vi "总氮通讯.vi"() -> ()   [LabVIEW 2016, in "斯坦道总氮.lvlib"]
uses:
  <vilib>/NI/Modbus Library/API/Wrapper/Create TCP Slave.vi
  <vilib>/Utility/config.llb/Write Key (Boolean).vi
  <vilib>/Utility/config.llb/Write Key (String).vi
  <vilib>/Plasmionique/MB Master/MB_Master/MB_Master.lvclass
  <vilib>/NI/Modbus Library/API/Slave/Modbus Slave.lvclass
  <vilib>/Utility/config.llb/NI_LVConfig.lvlib
  <vilib>/Plasmionique/MB Master/MB Master.lvlib
  <vilib>/NI/Modbus Library/API/Wrapper/API Main.lvlib
panel:
  out "总氮测量数据区":u16[](array[numeric])
  out "总氮状态告警区":u16[](array[numeric])
  out "总磷状态告警区":u16[](array[numeric])
  out "总磷测量数据区":u16[](array[numeric])
  out "序列号":string
  out "状态告警区":T1 {"告警代码" items=["无告警", "缺试剂告警", "缺水样告警", "缺蒸馏水告警", "缺标液告警", "仪表漏液告警", "标定异常告警", "超量程告警", "加热异常", "低试剂预警", "超上限告警", "超下限告警", "仪表内部其他异常", "滴定异常告警", "电极异常告警", "量程切换告警", "参数设置告警", "PH电极电位异常", "电导率电极异常", "浊度光度异常", "溶解氧电极异常", "溶解氧光强异常", "温度异常告警", "PH异常告警", "溶解氧异常告警", "电导率异常告警", "浊度异常告警", "叶绿素异常告警", "藻密度异常告警", "蓝绿藻异常告警", "ORP异常告警", "氨氮异常告警", "清洁刷异常告警", "SD卡异常告警", "蓝牙异常告警", "Wifi异常告警", "流程异常告警"]; "故障代码" items=["无故障", "电机故障", "温度故障", "通讯故障", "滴定故障"]}
  out "测量数据区":T2 {"单位" items=["ug/L", "mg/L", "ppm", "mg/m3", "cm", "ppb", "ug/m3", "%", "nmol/mol", "umol/mol", "MPN/L", "MPN/100ml", "ng/m3", "NTU", "无量纲", "ms/cm", "us/cm", "℃", "mV", "万个/L"]}
  out "status":bool
  out "关键参数区":T3
  in  "读关键参数区":bool
  in  "读状态告警区":bool
  in  "读测量数据区":bool
  in  "站号":u16(ring) items=["总磷"=1, "氨氮"=3]
  in  "停止":bool
  in  "启动":bool
  in  "控制命令":u16(ring) items=["启动测量"=1, "标样核查"=2, "零点核查"=3, "跨度核查"=4, "空白测试"=5, "平行样测试"=6, "加标回收"=7, "空白校准"=8, "标样校准"=9, "初始化（清洗）"=10, "停止测试"=11, "仪器重启"=12, "校时"=13, "模式设置"=14, "测量间隔设置"=15]
  in  "控制命令参数":u16[](array[numeric]) format="%04xH"
  in  "VISA Resource":refnum<visa-resource-name>
  in  "启用模块":bool
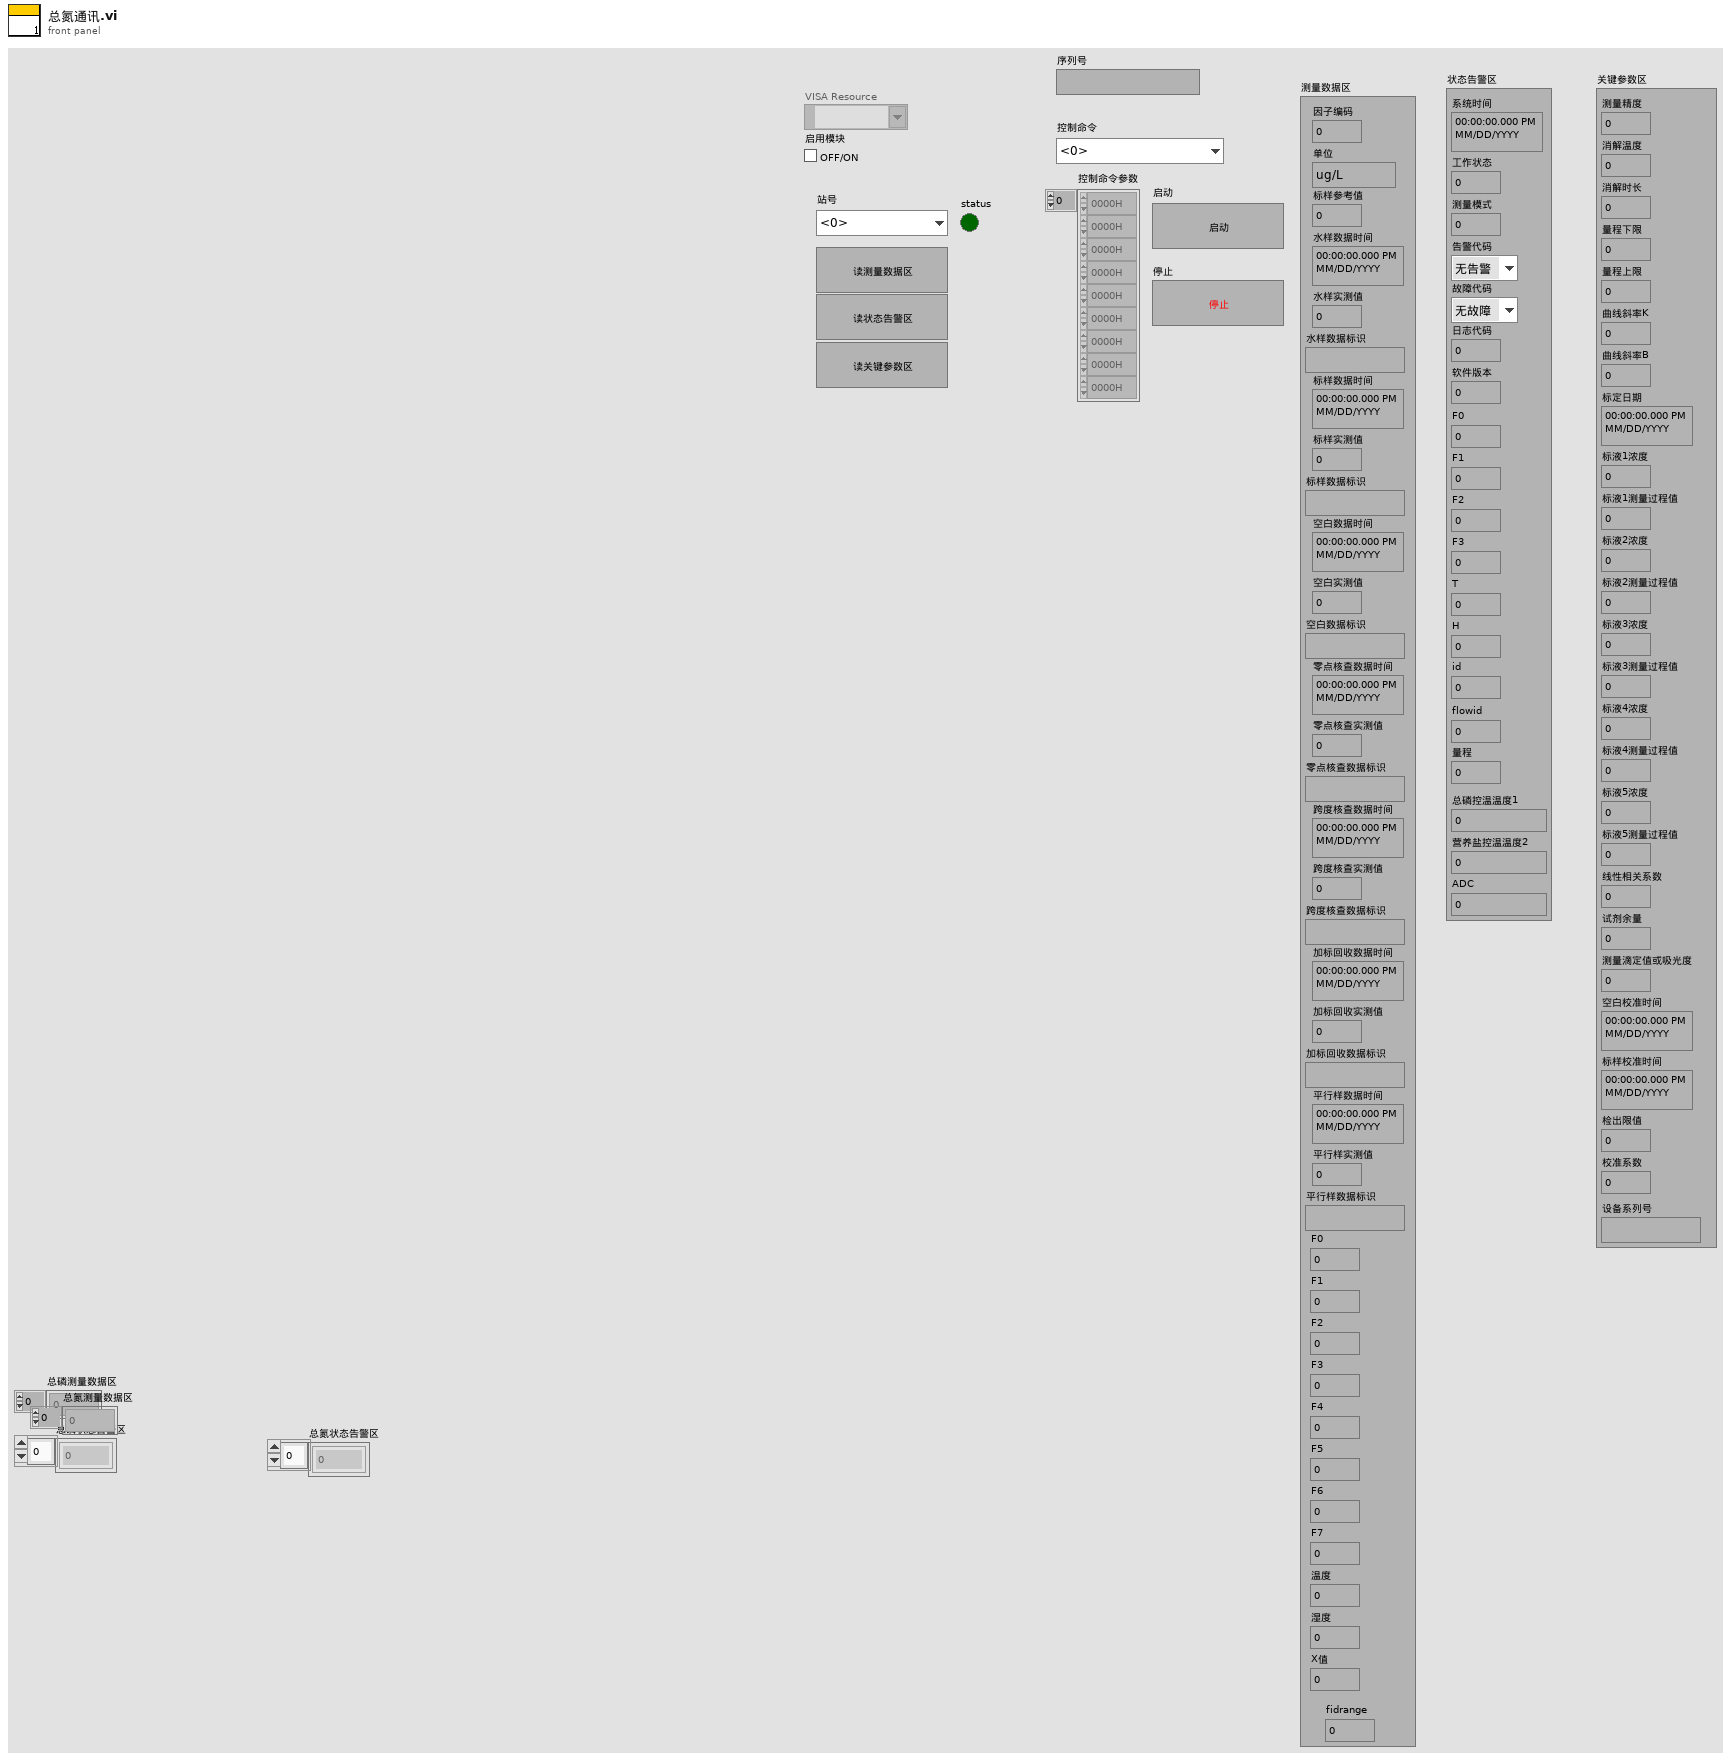
[diagram p1: front panel]
types:
  T1 = cluster{"系统时间":timestamp, "工作状态":u16, "测量模式":u16, "告警代码":u16, "故障代码":u16, "日志代码":u16, "软件版本":u16, "F0":sgl, "F1":sgl, "F2":sgl, "F3":sgl, "T":sgl, "H":sgl, "id":u16, "flowid":u16, "量程":u16, "总磷控温温度1":sgl, "营养盐控温温度2":sgl, "ADC":sgl}
  T2 = cluster{"因子编码":u32, "单位":u16, "标样参考值":sgl, "水样数据时间":timestamp, "水样实测值":sgl, "水样数据标识":string, "标样数据时间":timestamp, "标样实测值":sgl, "标样数据标识":string, "空白数据时间":timestamp, "空白实测值":sgl, "空白数据标识":string, "零点核查数据时间":timestamp, "零点核查实测值":sgl, "零点核查数据标识":string, "跨度核查数据时间":timestamp, "跨度核查实测值":sgl, "跨度核查数据标识":string, "加标回收数据时间":timestamp, "加标回收实测值":sgl, "加标回收数据标识":string, "平行样数据时间":timestamp, "平行样实测值":sgl, "平行样数据标识":string, "F0":sgl, "F1":sgl, "F2":sgl, "F3":sgl, "F4":sgl, "F5":sgl, "F6":sgl, "F7":sgl, "温度":sgl, "湿度":sgl, "X值":sgl, "fidrange":u16}
  T3 = cluster{"测量精度":u16, "消解温度":u16, "消解时长":u16, "量程下限":sgl, "量程上限":sgl, "曲线斜率K":sgl, "曲线斜率B":sgl, "标定日期":timestamp, "标液1浓度":sgl, "标液1测量过程值":sgl, "标液2浓度":sgl, "标液2测量过程值":sgl, "标液3浓度":sgl, "标液3测量过程值":sgl, "标液4浓度":sgl, "标液4测量过程值":sgl, "标液5浓度":sgl, "标液5测量过程值":sgl, "线性相关系数":sgl, "试剂余量":u32, "测量滴定值或吸光度":sgl, "空白校准时间":timestamp, "标样校准时间":timestamp, "检出限值":sgl, "校准系数":sgl, "设备系列号":string}
  T4 = typedef "NI_LVConfig.lvlib/Config Data RefNum.ctl" = refnum<k1>
  T5 = enum8{"Enabled", "Disabled", "Disabled and Grayed Out"}
  T6 = cluster{"系统时间":timestamp, "工作状态":enum16{"空闲", "水样测试", "标样核查", "零点核查", "跨度核查", "空白测试", "平行样测试", "加标回收", "空白校准", "标样校准", "初始化（清洗）"}, "测量模式":enum16{"待机", "连续模式", "周期模式", "定点模式", "受控模式", "手动模式"}, "告警代码":u16, "故障代码":u16, "日志代码":u16, "软件版本":u16, "F0":sgl, "F1":sgl, "F2":sgl, "F3":sgl, "T":sgl, "H":sgl, "id":u16, "flowid":u16, "量程":u16, "总磷控温温度1":sgl, "营养盐控温温度2":sgl, "ADC":sgl}
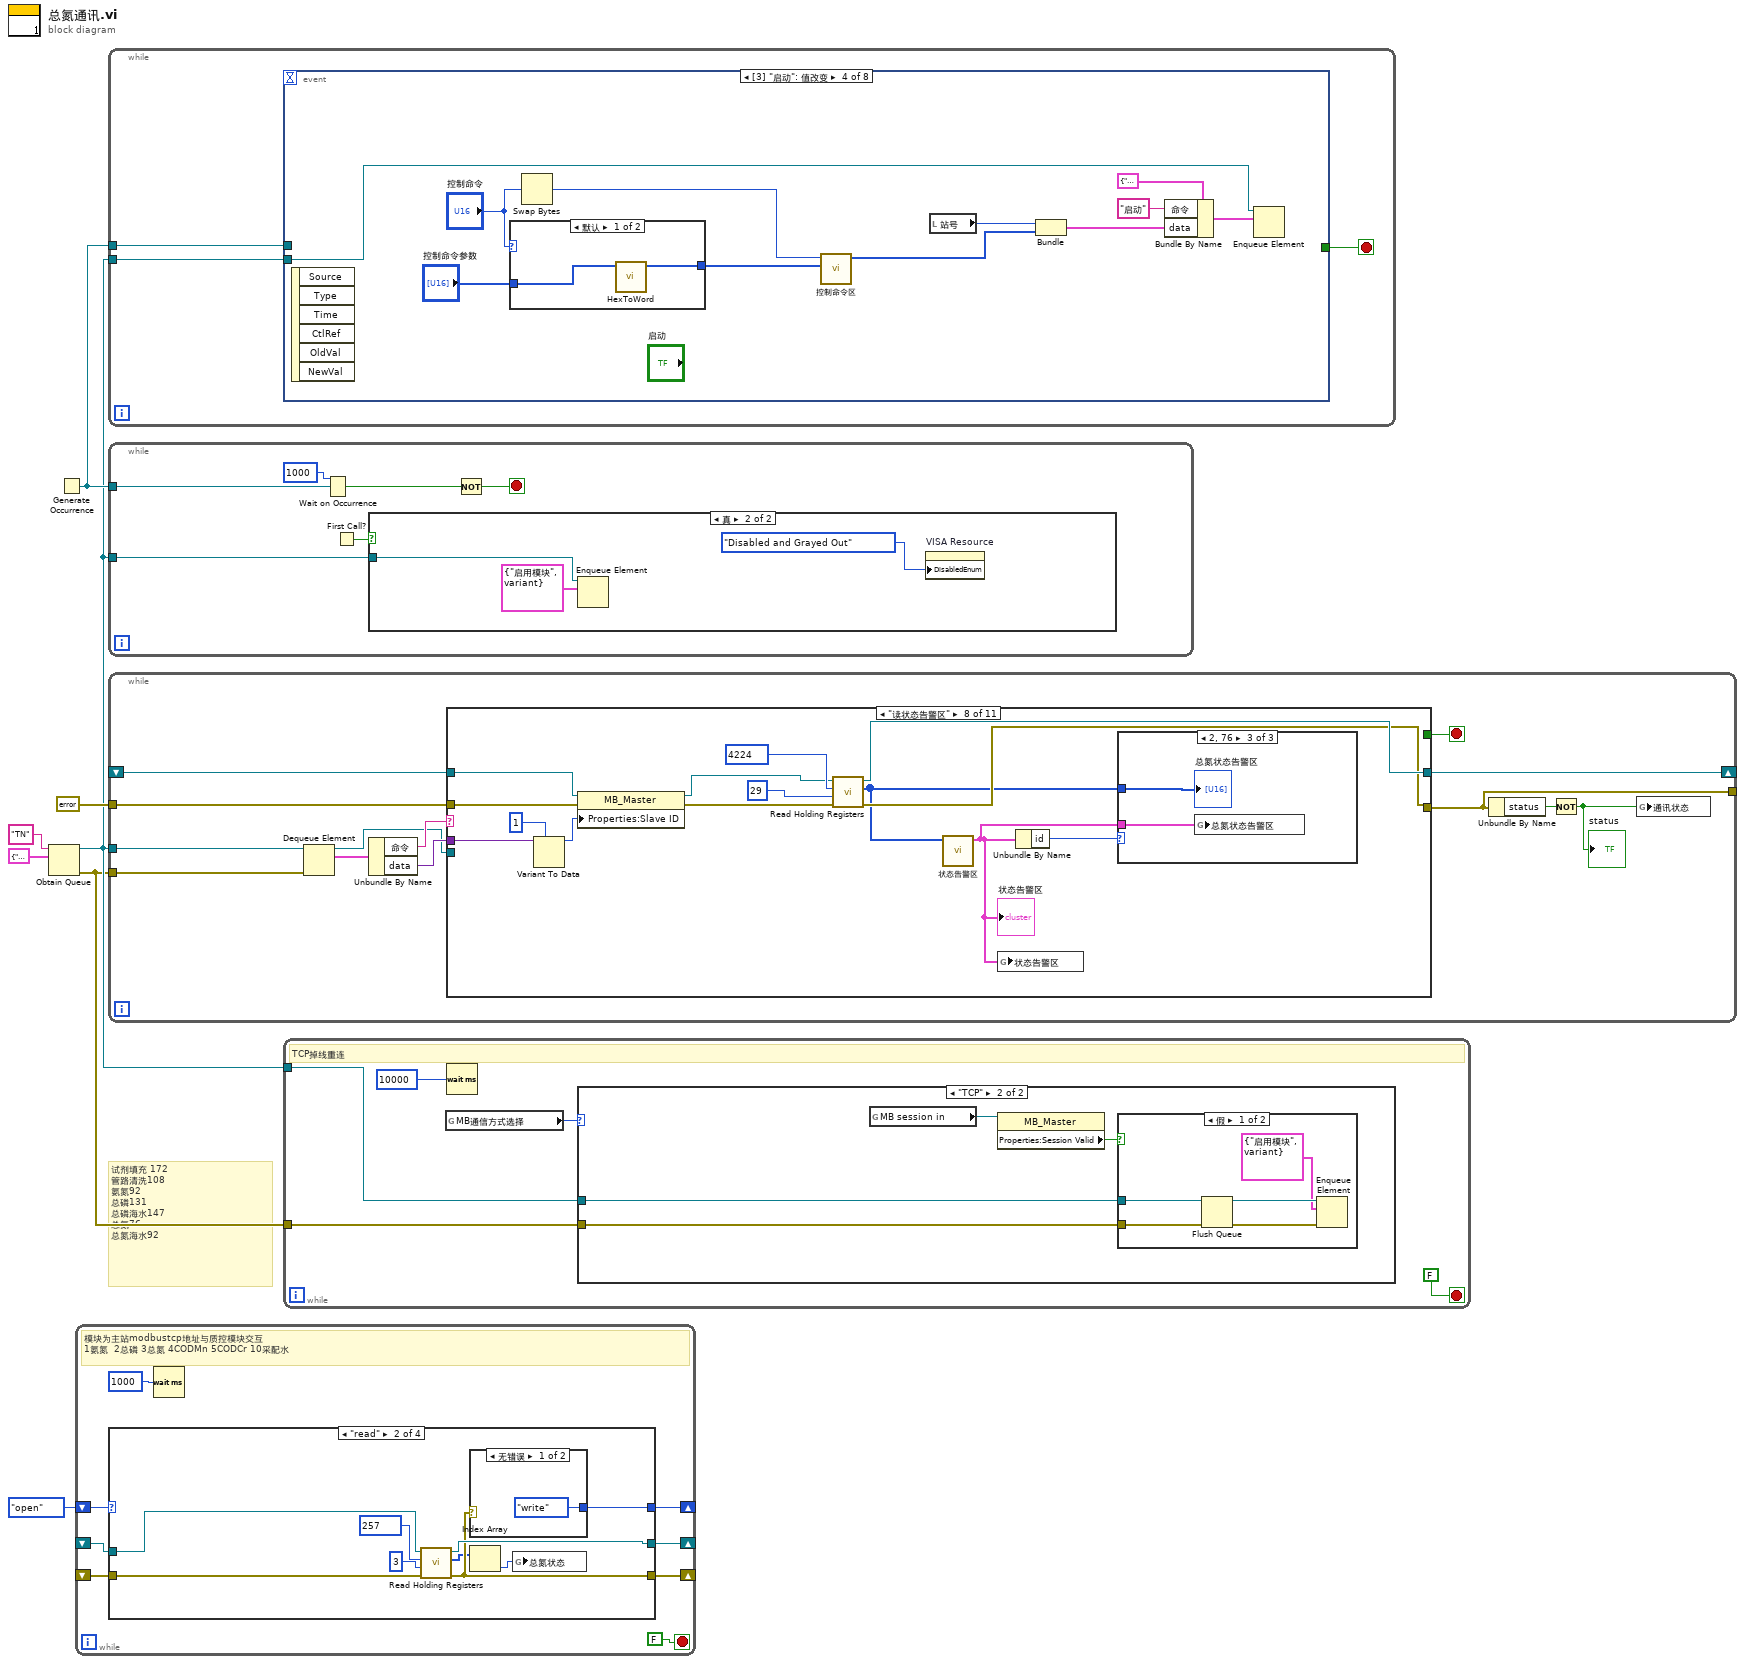
[diagram p0: block diagram]
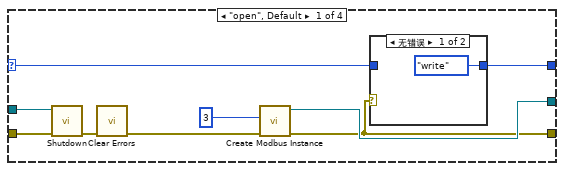
[diagram p4: hidden frame]
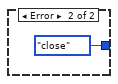
[diagram p6: hidden frame]
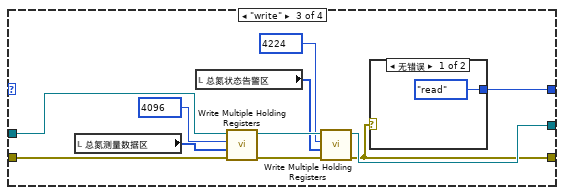
[diagram p7: hidden frame]
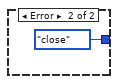
[diagram p8: hidden frame]
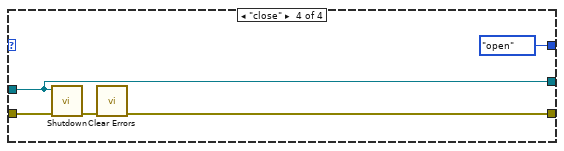
[diagram p9: hidden frame]
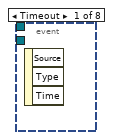
[diagram p11: hidden frame]
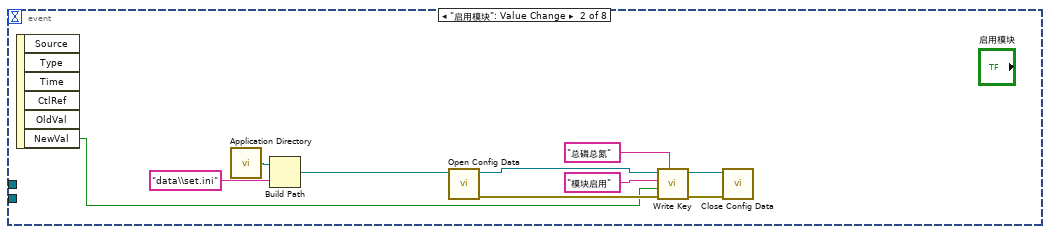
[diagram p12: hidden frame]
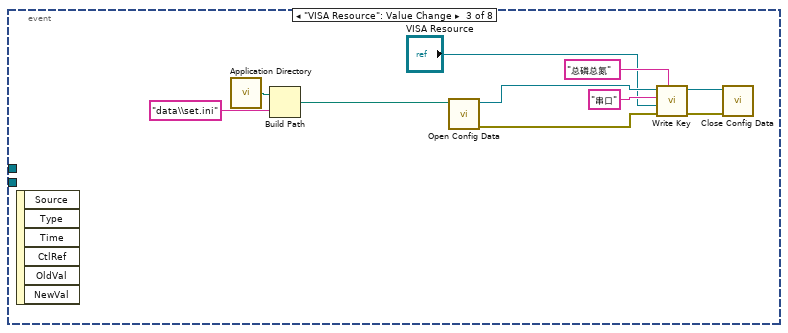
[diagram p13: hidden frame]
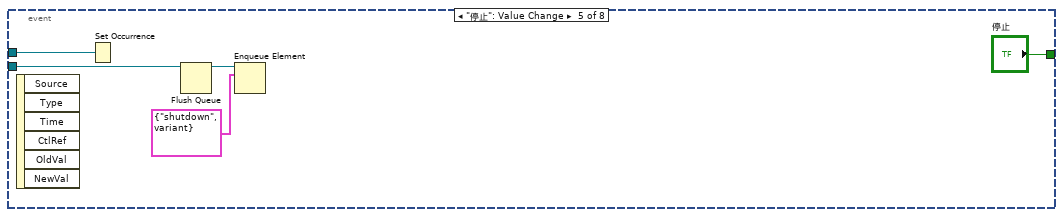
[diagram p15: hidden frame]
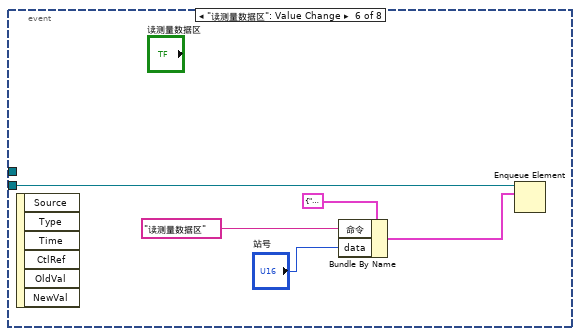
[diagram p16: hidden frame]
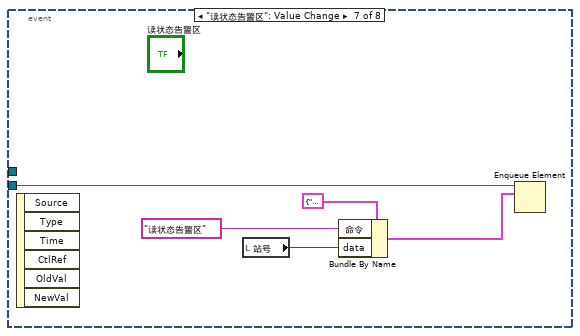
[diagram p17: hidden frame]
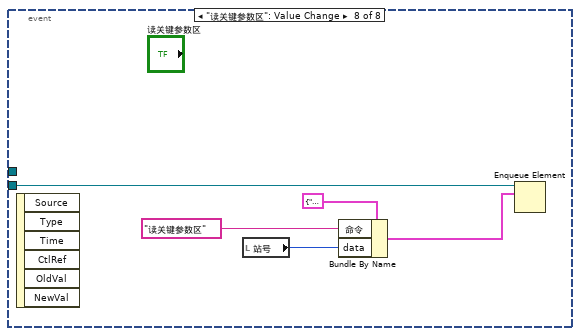
[diagram p18: hidden frame]
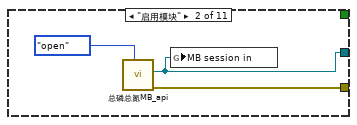
[diagram p20: hidden frame]
diagram:
  # "试剂填充 172 \n管路清洗108\n氨氮92\n总磷131\n总磷海水147\n总氮76\n总氮海水92"
  n1 = Obtain Queue(name (unnamed)="TN" ("名称（未命名）"), element data type=cluster{"命令":string, "data":variant} {"命令"="", "data"=variant}) -> (queue out=w2:refnum<queue>, error out=w1:errorcluster)  [unwired: 3 in, 1 out]
  n2 = Generate Occurrence() -> (w4:refnum<k4>)
  n3 = while {
    shift-right: [w13] -> _
    shift-left: _ -> [w15]
    shift-right: [w12] -> _
    shift-left: _ -> [w14]
    shift-right: [w9] -> _
    shift-left: enum16{"open", "read", "write", "close"}."open" -> [w10]
    stop <- FALSE stop-if-true
    # "模块为主站modbustcp地址与质控模块交互\n1氨氮  2总磷 3总氮 4CODMn 5CODCr 10采配水"
    n4 = case shown="\"read\"" w10 {
      selector: w10 -> [w24 _ _ _]
      tunnel: w15 -> [w18 w34 w47 w53]
      tunnel: w14 -> [w17 w33 w46 w52]
      tunnel: [w21 w30 w42 w53] -> w13
      tunnel: [w20 w29 w41 w55] -> w12
      tunnel: [w23 w35 w48 enum16{"open", "read", "write", "close"}."open"] -> w9
      frame "open", Default {
        n5 = call-dynamic "Shutdown.vi"("error in"=w17, "Modbus slave in"=w18) -> ("error out"=w16:errorcluster)  [unwired: 9 in]
        n6 = call <vilib>:"Clear Errors.vi"("error in (no error)"=w16) -> ("error out"=w19:errorcluster)  [unwired: 5 in, 1 out]
        n7 = call-poly <vilib>:"Create Modbus Instance.vi"("error in"=w19, "port (502)"=u16 3) -> ("error out"=w20:errorcluster, "TCP slave instance"=w21:refnum<class "Modbus Slave.lvclass">)  [unwired: 8 in]
        n8 = case shown="无错误" w20 {
          tunnel: w24 -> [_ w26]
          tunnel: [enum16{"open", "read", "write", "close"}."write" w26] -> w23
          frame No Error {
          }
          frame Error {
          }
        }
      }
      frame "read" {
        n9 = call-dynamic <vilib>:"Read Holding Registers.vi"("error in"=w33, "number of inputs"=u16 3, "starting address"=u16 257, "Modbus slave in"=w34) -> ("error out"=w29:errorcluster, "register values"=w28:u16[], "Modbus slave out"=w30:refnum<class "Modbus Slave.lvclass">)  [unwired: 5 in]
        n10 = case shown="无错误" w29 {
          tunnel: [enum16{"open", "read", "write", "close"}."write" enum16{"open", "read", "write", "close"}."close"] -> w35
          frame No Error {
          }
          frame Error {
          }
        }
        n11 = Index Array(array=w28) -> (element=w27:u16)  [unwired: 1 in]
        n12 = global write "VAR总氮全局变量.vi" "总氮状态"(w27) -> ()
      }
      frame "write" {
        n13 = local read "总氮测量数据区"() -> (w40:u16[])
        n14 = local read "总氮状态告警区"() -> (w38:u16[])
        n15 = call-dynamic "Write Multiple Holding Registers.vi"("error in"=w46, "registers to write"=w40, "starting address"=u16 4096, "Modbus slave in"=w47) -> ("error out"=w43:errorcluster, "Modbus slave out"=w44:refnum<class "Modbus Slave.lvclass">)  [unwired: 6 in]
        n16 = call-dynamic "Write Multiple Holding Registers.vi"("error in"=w43, "registers to write"=w38, "starting address"=u16 4224, "Modbus slave in"=w44) -> ("error out"=w41:errorcluster, "Modbus slave out"=w42:refnum<class "Modbus Slave.lvclass">)  [unwired: 6 in]
        n17 = case shown="无错误" w41 {
          tunnel: [enum16{"open", "read", "write", "close"}."read" enum16{"open", "read", "write", "close"}."close"] -> w48
          frame No Error {
          }
          frame Error {
          }
        }
      }
      frame "close" {
        n18 = call-dynamic "Shutdown.vi"("error in"=w52, "Modbus slave in"=w53) -> ("error out"=w51:errorcluster)  [unwired: 9 in]
        n19 = call <vilib>:"Clear Errors.vi"("error in (no error)"=w51) -> ("error out"=w55:errorcluster)  [unwired: 5 in, 1 out]
      }
    }
    n20 = Wait (ms)(milliseconds to wait=u32 1000 ("等待时间（毫秒）")) -> ()  [unwired: 1 out]
  }
  n21 = while {
    tunnel: w2 -> [w58]
    tunnel: w4 -> [w56]
    stop <- w57 stop-if-true
    n22 = event shown="[3] \"启动\": 值改变" {
      selector: _ -> [_ _ _ _ _ _ _ _]
      dyn-events: _ -> [_ _ _ _ _ _ _ _]
      timeout: _ -> [_ _ _ _ _ _ _ _]
      tunnel: w58 -> [_ _ _ w89 w96 w102 w107 w112]
      tunnel: [_ _ _ _ "停止" _ _ _] -> w57
      tunnel: w56 -> [_ _ _ _ w93 _ _ _]
      event Timeout {
        n23 = event-data() -> ()  [unwired: 1 in, 3 out]
      }
      event "启用模块": Value Change {
        n24 = event-data() -> ("NewVal"=w59:bool)  [unwired: 1 in, 5 out]
        n25 = call <vilib>:"Application Directory.vi"() -> ("Application Directory"=w61:path)
        n26 = Build Path(base path=w61, name or relative path="data\\set.ini" ("名称或相对路径")) -> (appended path=w62:path)
        n27 = call <vilib>:"Open Config Data.vi"("configuration file path"=w62) -> ("error out"=w68:errorcluster, "refnum"=w67:T4)  [unwired: 8 in, 1 out]
        n28 = call-poly <vilib>:"Write Key.vi"("section"="总磷总氮", "error in (no error)"=w68, "value"=w59, "key"="模块启用", "refnum"=w67) -> ("error out"=w64:errorcluster, "refnum out"=w60:T4)  [unwired: 4 in, 1 out]
        n29 = call <vilib>:"Close Config Data.vi"("error in (no error)"=w64, "refnum"=w60) -> ()  [unwired: 8 in, 2 out]
      }
      event "VISA Resource": Value Change {
        n30 = event-data() -> ()  [unwired: 1 in, 6 out]
        n31 = call <vilib>:"Application Directory.vi"() -> ("Application Directory"=w71:path)
        n32 = Build Path(base path=w71, name or relative path="data\\set.ini" ("名称或相对路径")) -> (appended path=w72:path)
        n33 = call <vilib>:"Open Config Data.vi"("configuration file path"=w72) -> ("error out"=w78:errorcluster, "refnum"=w77:T4)  [unwired: 8 in, 1 out]
        n34 = call-poly <vilib>:"Write Key.vi"("section"="总磷总氮", "error in (no error)"=w78, "value"="VISA Resource", "key"="串口", "refnum"=w77) -> ("error out"=w74:errorcluster, "refnum out"=w70:T4)  [unwired: 4 in, 1 out]
        n35 = call <vilib>:"Close Config Data.vi"("error in (no error)"=w74, "refnum"=w70) -> ()  [unwired: 8 in, 2 out]
      }
      event "启动": Value Change {
        n36 = event-data() -> ()  [unwired: 1 in, 6 out]
        n37 = case shown="默认" "控制命令" {
          tunnel: "控制命令参数" -> [w91 w92]
          tunnel: [w90 w92] -> w79
          frame Default {
            n38 = call "HexToWord.vi"("数组"=w91) -> ("WORD"=w90:u16[])  [unwired: 10 in]
          }
          frame 13 {
          }
        }
        n39 = Swap Bytes(anything="控制命令") -> (byte swapped=w82:u16)
        n40 = call "控制命令区.vi"("控制命令参数"=w79, "控制命令"=w82) -> ("控制命令"=w85:u16[])  [unwired: 9 in]
        n41 = local read "站号"() -> (w84:u16)
        n42 = Bundle("站号"=w84, "控制命令"=w85) -> (w83:cluster{"站号":u16, "控制命令":u16[]})  [unwired: 1 in]
        n43 = Bundle By Name(cluster=cluster{"命令":string, "data":variant} {"命令"="", "data"=variant} ("元素"), "命令"="启动", "data"=w83) -> (w87:cluster{"命令":string, "data":variant})
        n44 = Enqueue Element(queue=w89, element=w87) -> ()  [unwired: 2 in, 3 out]
      }
      event "停止": Value Change {
        n45 = event-data() -> ()  [unwired: 1 in, 6 out]
        n46 = Set Occurrence(w93) -> ()
        n47 = Flush Queue(queue=w96) -> (queue out=w95:refnum<queue>)  [unwired: 1 in, 2 out]
        n48 = Enqueue Element(queue=w95, element=cluster{"命令":string, "data":variant} {"命令"="shutdown", "data"=variant} ("元素")) -> ()  [unwired: 2 in, 3 out]
      }
      event "读测量数据区": Value Change {
        n49 = event-data() -> ()  [unwired: 1 in, 6 out]
        n50 = Bundle By Name(cluster=cluster{"命令":string, "data":variant} {"命令"="", "data"=variant} ("元素"), "命令"="读测量数据区", "data"="站号") -> (w100:cluster{"命令":string, "data":variant})
        n51 = Enqueue Element(queue=w102, element=w100) -> ()  [unwired: 2 in, 3 out]
      }
      event "读状态告警区": Value Change {
        n52 = event-data() -> ()  [unwired: 1 in, 6 out]
        n53 = local read "站号"() -> (w103:u16)
        n54 = Bundle By Name(cluster=cluster{"命令":string, "data":variant} {"命令"="", "data"=variant} ("元素"), "命令"="读状态告警区", "data"=w103) -> (w105:cluster{"命令":string, "data":variant})
        n55 = Enqueue Element(queue=w107, element=w105) -> ()  [unwired: 2 in, 3 out]
      }
      event "读关键参数区": Value Change {
        n56 = event-data() -> ()  [unwired: 1 in, 6 out]
        n57 = local read "站号"() -> (w108:u16)
        n58 = Bundle By Name(cluster=cluster{"命令":string, "data":variant} {"命令"="", "data"=variant} ("元素"), "命令"="读关键参数区", "data"=w108) -> (w110:cluster{"命令":string, "data":variant})
        n59 = Enqueue Element(queue=w112, element=w110) -> ()  [unwired: 2 in, 3 out]
      }
    }
  }
  n60 = while {
    tunnel: w4 -> [w118]
    tunnel: w2 -> [w114]
    stop <- w115 stop-if-true
    n61 = Wait on Occurrence(2:w118, 3:1000 ("毫秒超时(-1)")) -> (0:w116:bool)  [unwired: 1 in]
    n62 = First Call?() -> (First Call?: T/F=w113:bool)
    n63 = case shown="真" w113 {
      tunnel: w114 -> [_ w120]
      frame False {
      }
      frame True {
        n64 = Enqueue Element(queue=w120, element=cluster{"命令":string, "data":variant} {"命令"="启用模块", "data"=variant} ("元素")) -> ()  [unwired: 2 in, 3 out]
        n65 = property on="VISA Resource" class="VISAName"("DisabledEnum"=T5."Disabled and Grayed Out" ("禁用")) -> ()  [unwired: 2 in, 2 out]
      }
    }
    n66 = Not(x=w116) -> (.not. x?=w115:bool)
  }
  n67 = while {
    tunnel: w2 -> [w134]
    tunnel: w1 -> [w133]
    shift-right: [w131] -> _
    shift-left: _ -> [w130]
    tunnel: errorcluster {"status"=FALSE, "code"=0, "source"=""} ("error out") -> [w129]
    tunnel: [w124] -> _
    stop <- w132 stop-if-true
    n68 = Dequeue Element(queue=w134, error in (no error)=w133) -> (queue out=w125:refnum<queue>, element=w127:cluster{"命令":string, "data":variant})  [unwired: 1 in, 2 out]
    n69 = Unbundle By Name(w127) -> ("命令"=w128:string, "data"=w126:variant)
    n70 = case shown="\"读状态告警区\"" w128 {
      tunnel: w126 -> [_ _ _ w153 w164 w181 w191 w205 w223 w237 _]
      tunnel: w125 -> [_ _ _ _ _ _ _ _ _ _ w250]
      tunnel: [_ _ _ _ _ _ _ _ _ _ TRUE] -> w132
      tunnel: [w135 w138 w140 w156 w167 w183 w195 w214 w230 w244 w246] -> w131
      tunnel: [w136 w137 w141 w155 w166 w182 w196 w204 w231 w245 w247] -> w124
      tunnel: w130 -> [w135 _ w140 w152 w163 w180 w190 w208 w226 w240 w246]
      tunnel: w129 -> [w136 _ w143 w149 w160 w177 w188 w209 w227 w241 w248]
      frame Default {
      }
      frame "启用模块" {
        n71 = call "总磷总氮MB_api.vi"("STEP"=enum16{"open", "read", "write", "close"}."open") -> ("error out"=w137:errorcluster, "MB session out"=w138:refnum<class "MB_Master.lvclass">)  [unwired: 8 in, 1 out]
        n72 = global write "VAR总氮全局变量.vi" "MB session in"(w138) -> ()
      }
      frame "停用模块" {
        n73 = call-dynamic "Close Session.vi"("error in (no error)"=w143, "MB session in"=w140) -> ("error out"=w142:errorcluster)  [unwired: 9 in]
        n74 = call <vilib>:"Clear Errors.vi"("error in (no error)"=w142) -> ("error out"=w141:errorcluster)  [unwired: 5 in, 1 out]
      }
      frame "启动" {
        n75 = Variant To Data(type=cluster{"站号":u16, "控制命令":u16[]} {"站号"=0, "控制命令"=[]} ("输出簇"), Variant=w153) -> (data=w147:cluster{"站号":u16, "控制命令":u16[]})  [unwired: 1 in, 1 out]
        n76 = Unbundle By Name(w147) -> ("站号"=w146:u16, "控制命令"=w144:u16[])
        n77 = property class="MB_Master"(reference=w152, error in=w149, "Properties:Slave ID"=w146) -> (reference out=w151:refnum<class "MB_Master.lvclass">, error out=w150:errorcluster)
        n78 = Index Array(array=w144) -> (element=w145:u16)  [unwired: 1 in]
        n79 = global write "VAR总氮全局变量.vi" "控制命令"(w145) -> ()
        n80 = call <vilib>:"Write Multiple Registers.vi"("error in (no error)"=w150, "values"=w144, "starting address"=u16 4608, "MB session in"=w151) -> ("error out"=w155:errorcluster, "MB session out"=w156:refnum<class "MB_Master.lvclass">)  [unwired: 6 in]
      }
      frame "盲样测试" {
        n81 = Variant To Data(type=0, Variant=w164) -> (data=w157:i32)  [unwired: 1 in, 1 out]
        n82 = property class="MB_Master"(reference=w163, error in=w160, "Properties:Slave ID"=w157) -> (reference out=w162:refnum<class "MB_Master.lvclass">, error out=w161:errorcluster)
        n83 = case shown="默认" w157 {
          tunnel: [u16[] [] ("values") u16[] [33539, 0] ("values") u16[] [23555, 0] ("values")] -> w159
          frame Default {
          }
          frame 1 {
            # "总磷盲样测试命令"
          }
          frame 3 {
            # "氨氮盲样测试"
          }
        }
        n84 = call <vilib>:"Write Multiple Registers.vi"("error in (no error)"=w161, "values"=w159, "starting address"=u16 24592, "MB session in"=w162) -> ("error out"=w166:errorcluster, "MB session out"=w167:refnum<class "MB_Master.lvclass">)  [unwired: 6 in]
      }
      frame "debug" {
        n85 = Variant To Data(type=cluster{"站号":u16, "控制命令":u16[]} {"站号"=0, "控制命令"=[]} ("输出簇"), Variant=w181) -> (data=w175:cluster{"站号":u16, "控制命令":u16[]})  [unwired: 1 in, 1 out]
        n86 = Unbundle By Name(w175) -> ("站号"=w174:u16, "控制命令"=w172:u16[])
        n87 = property class="MB_Master"(reference=w180, error in=w177, "Properties:Slave ID"=w174) -> (reference out=w179:refnum<class "MB_Master.lvclass">, error out=w178:errorcluster)
        n88 = Index Array(array=w172) -> (element=w173:u16)  [unwired: 1 in]
        n89 = global write "VAR总氮全局变量.vi" "控制命令"(w173) -> ()
        n90 = call <vilib>:"Write Multiple Registers.vi"("error in (no error)"=w178, "values"=w172, "starting address"=u16 24594, "MB session in"=w179) -> ("error out"=w182:errorcluster, "MB session out"=w183:refnum<class "MB_Master.lvclass">)  [unwired: 6 in]
      }
      frame "读测量数据区" {
        n91 = Variant To Data(type=u8 1 ("Slave ID"), Variant=w191) -> (data=w186:u8)  [unwired: 1 in, 1 out]
        n92 = property class="MB_Master"(reference=w190, error in=w188, "Properties:Slave ID"=w186) -> (reference out=w189:refnum<class "MB_Master.lvclass">, error out=w187:errorcluster)
        n93 = call <vilib>:"Read Holding Registers.vi"("error in (no error)"=w187, "quantity"=u16 105, "starting address"=u16 4096, "MB session in"=w189) -> ("error out"=w196:errorcluster, "Registers"=w185:u16[], "MB session out"=w195:refnum<class "MB_Master.lvclass">)  [unwired: 5 in]
        n94 = call "测量数据区.vi"("数组"=w185) -> ("测量数据区"=w184:T2)  [unwired: 10 in]
        "测量数据区" <- w184
        n95 = global write "VAR总氮全局变量.vi" "测量数据区"(w184) -> ()
        n96 = case shown="2" w186 {
          tunnel: w184 -> [_ w197 w199]
          tunnel: w185 -> [_ w198 w200]
          frame 0, Default {
          }
          frame 1 {
            n97 = global write "VAR总氮全局变量.vi" "总磷测量数据区"(w197) -> ()
            "总磷测量数据区" <- w198
          }
          frame 2 {
            n98 = global write "VAR总氮全局变量.vi" "总氮测量数据区"(w199) -> ()
            "总氮测量数据区" <- w200
          }
        }
      }
      frame "读状态告警区" {
        n99 = Variant To Data(type=u8 1 ("Slave ID"), Variant=w205) -> (data=w210:u8)  [unwired: 1 in, 1 out]
        n100 = property class="MB_Master"(reference=w208, error in=w209, "Properties:Slave ID"=w210) -> (reference out=w207:refnum<class "MB_Master.lvclass">, error out=w206:errorcluster)
        n101 = call <vilib>:"Read Holding Registers.vi"("error in (no error)"=w206, "quantity"=u16 29, "starting address"=u16 4224, "MB session in"=w207) -> ("error out"=w204:errorcluster, "Registers"=w201:u16[], "MB session out"=w214:refnum<class "MB_Master.lvclass">)  [unwired: 5 in]
        n102 = call "状态告警区.vi"("数组"=w201) -> ("状态告警区"=w202:T6)  [unwired: 10 in]
        "状态告警区" <- w202
        n103 = global write "VAR总氮全局变量.vi" "状态告警区"(w202) -> ()
        n104 = Unbundle By Name(w202) -> ("id"=w203:u16)
        n105 = case shown="2, 76" w203 {
          tunnel: w202 -> [_ w215 w217]
          tunnel: w201 -> [_ w216 w218]
          frame 0, Default {
          }
          frame 1, 131 {
            n106 = global write "VAR总氮全局变量.vi" "总磷状态告警区"(w215) -> ()
            "总磷状态告警区" <- w216
          }
          frame 2, 76 {
            n107 = global write "VAR总氮全局变量.vi" "总氮状态告警区"(w217) -> ()
            "总氮状态告警区" <- w218
          }
        }
      }
      frame "读关键参数区" {
        n108 = Variant To Data(type=u8 1 ("Slave ID"), Variant=w223) -> (data=w221:u8)  [unwired: 1 in, 1 out]
        n109 = property class="MB_Master"(reference=w226, error in=w227, "Properties:Slave ID"=w221) -> (reference out=w225:refnum<class "MB_Master.lvclass">, error out=w224:errorcluster)
        n110 = call <vilib>:"Read Holding Registers.vi"("error in (no error)"=w224, "quantity"=u16 19, "starting address"=u16 4256, "MB session in"=w225) -> ("error out"=w231:errorcluster, "Registers"=w220:u16[], "MB session out"=w230:refnum<class "MB_Master.lvclass">)  [unwired: 5 in]
        n111 = call "关键参数区.vi"("数组"=w220) -> ("关键参数区"=w219:T3)  [unwired: 10 in]
        "关键参数区" <- w219
        n112 = global write "VAR总氮全局变量.vi" "关键参数区"(w219) -> ()
      }
      frame "读序列号" {
        n113 = Variant To Data(type=u8 1 ("Slave ID"), Variant=w237) -> (data=w235:u8)  [unwired: 1 in, 1 out]
        n114 = property class="MB_Master"(reference=w240, error in=w241, "Properties:Slave ID"=w235) -> (reference out=w239:refnum<class "MB_Master.lvclass">, error out=w238:errorcluster)
        n115 = call <vilib>:"Read Holding Registers.vi"("error in (no error)"=w238, "quantity"=u16 6, "starting address"=u16 4, "MB session in"=w239) -> ("error out"=w245:errorcluster, "Registers"=w234:u16[], "MB session out"=w244:refnum<class "MB_Master.lvclass">)  [unwired: 5 in]
        n116 = call "HexToString.vi"("数组"=w234) -> ("STRING"=w233:string[])  [unwired: 10 in]
        n117 = Index Array(array=w233) -> (element=w232:string)  [unwired: 1 in]
        "序列号" <- w232
        n118 = global write "VAR总氮全局变量.vi" "序列号"(w232) -> ()
      }
      frame "shutdown" {
        n119 = call-dynamic "Close Session.vi"("error in (no error)"=w248, "MB session in"=w246) -> ("error out"=w247:errorcluster)  [unwired: 9 in]
        n120 = Flush Queue(queue=w250) -> (queue out=w249:refnum<queue>)  [unwired: 1 in, 2 out]
        n121 = Release Queue(queue=w249) -> ()  [unwired: 2 in, 3 out]
      }
    }
    n122 = Unbundle By Name(w124) -> ("status"=w123:bool)
    n123 = Not(x=w123) -> (.not. x?=w122:bool)
    "status" <- w122
    n124 = global write "VAR总氮全局变量.vi" "通讯状态"(w122) -> ()
  }
  n125 = while "While循环" {
    tunnel: w2 -> [w254]
    tunnel: w1 -> [w253]
    stop <- FALSE stop-if-true
    # "TCP掉线重连"
    n126 = global read "总氮断电保存全局变量.vi" "MB通信方式选择"() -> (w252:enum16{"串口", "TCP"})
    n127 = Wait (ms)(milliseconds to wait=u32 10000 ("等待时间（毫秒）")) -> ()  [unwired: 1 out]
    n128 = case shown="\"TCP\"" w252 {
      tunnel: w254 -> [_ w259]
      tunnel: w253 -> [_ w258]
      frame "串口", Default {
      }
      frame "TCP" {
        n129 = global read "VAR总氮全局变量.vi" "MB session in"() -> (w257:refnum<class "MB_Master.lvclass">)
        n130 = property class="MB_Master"(reference=w257) -> ("Properties:Session Valid"=w260:bool)  [unwired: 1 in, 2 out]
        n131 = case shown="假" w260 {
          tunnel: w259 -> [w263 _]
          tunnel: w258 -> [w262 _]
          frame False {
            n132 = Flush Queue(queue=w263, error in (no error)=w262) -> (queue out=w265:refnum<queue>, error out=w264:errorcluster)  [unwired: 1 out]
            n133 = Enqueue Element(queue=w265, element=cluster{"命令":string, "data":variant} {"命令"="启用模块", "data"=variant} ("元素"), error in (no error)=w264) -> ()  [unwired: 1 in, 3 out]
          }
          frame True {
          }
        }
      }
    }
  }
